vi "Script_Create.vi"(0 "reference in":refnum<class "Script.lvclass">, 1 "Full Command":string, 2 "Script Name":string, 3 "Log File":string, 4 "IP Address":string, 5 "Error In":errorcluster, 6 "Update Rate (ms)":i32, 8 "Console Listbox":refnum<vi>, 10 "Script Complete Event":refnum<user-event>) -> (14 "reference out":refnum<class "Script.lvclass">, 19 "Error Out":errorcluster)   [LabVIEW 2023, in "Script.lvclass"]
uses:
  Script.lvclass
  Script.lvclass/Script.ctl
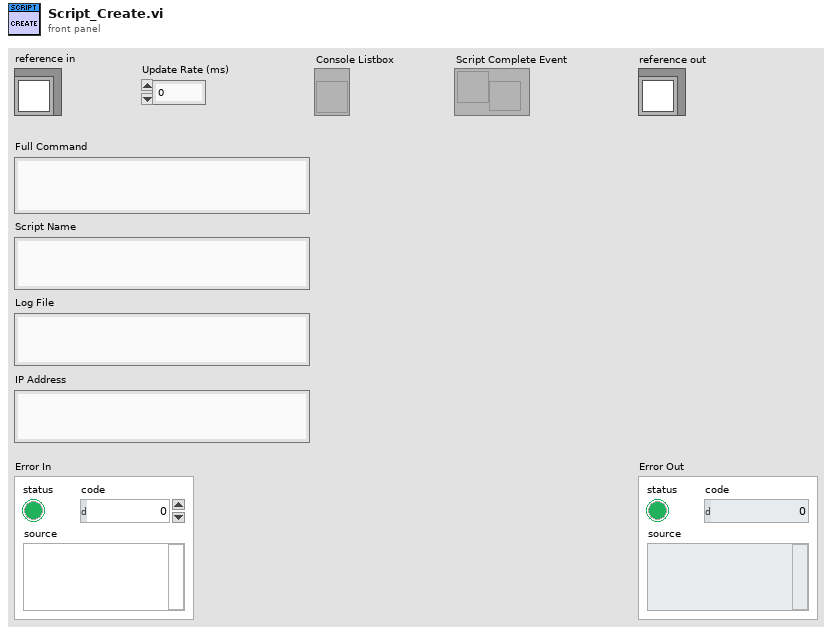
[diagram p1: front panel]
types:
  T1 = typedef "Script.lvclass/ObjectAttributes.ctl" = cluster{"Update Rate (ms)":i32, "Console Listbox":refnum<vi>, "Full Command":string, "Script Name":string, "Log File":string, "IP Address":string, "Script Complete Event":refnum<user-event>}
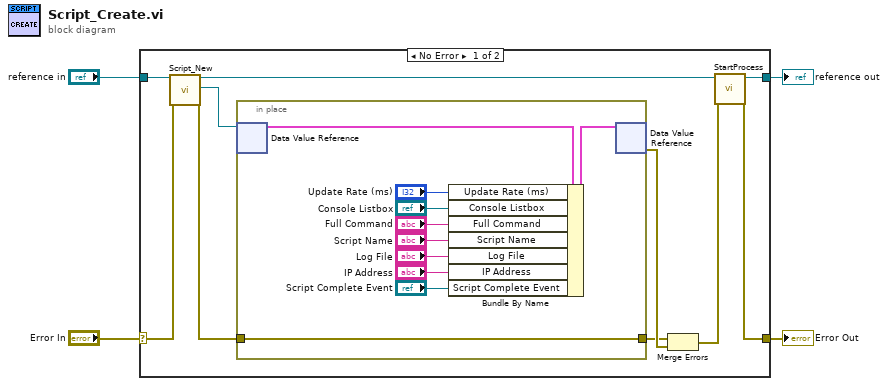
[diagram p0: block diagram]
diagram:
  n1 = case shown="No Error" "Error In" {
    selector: "Error In" -> [w13 w26]
    tunnel: [w5 w26] -> w3
    tunnel: "reference in" -> [w14 w25]
    tunnel: [w7 w25] -> w1
    frame No Error {
      n2 = call "Script_New.vi"("reference in"=w14, "Error In"=w13) -> ("reference out"=w8:refnum<class "Script.lvclass">, "DVRRefOut"=w11:refnum<data-value>, "Error Out"=w10:errorcluster)  [unwired: 14 in, 1 out]
      n3 = in-place {
        in-place-border: w10 -> [w22]
        in-place-border: [w22] -> w9
        n4 = in-place-dvr #1(w11) -> (w23:T1)  [unwired: 1 out]
        n5 = Bundle By Name(cluster=w23, "Update Rate (ms)"="Update Rate (ms)", "Console Listbox"="Console Listbox", "Full Command"="Full Command", "Script Name"="Script Name", "Log File"="Log File", "IP Address"="IP Address", "Script Complete Event"="Script Complete Event") -> (w24:T1)
        n6 = in-place-dvr #1(w24) -> (w12:errorcluster)  [unwired: 1 out]
      }
      n7 = Merge Errors(w9, w12) -> (w6:errorcluster)
      n8 = call "StartProcess.vi"("reference in"=w8, "Error In"=w6) -> ("reference out"=w7:refnum<class "Script.lvclass">, "Error Out"=w5:errorcluster)  [unwired: 14 in, 2 out]
    }
    frame Error {
      # "VI-TechBaseTemplate_Simple_6x8x6"
    }
  }
  "Error Out" <- w3
  "reference out" <- w1
